vi "CreateSyslog.vi"(6 "timestamp":timestamp, 7 "type":T1, 8 "error in":errorcluster, 10 "executiontime":dbl, 11 "log":string) -> (0 "error out":errorcluster, 3 "syslog out":refnum<class "syslogs.lvclass">)   [LabVIEW 2020, in "ORM_Examples.lvlib" / "syslogs.lvclass"]
uses:
  syslogs.lvclass
  type.ctl
  syslogs.lvclass/syslogs.ctl
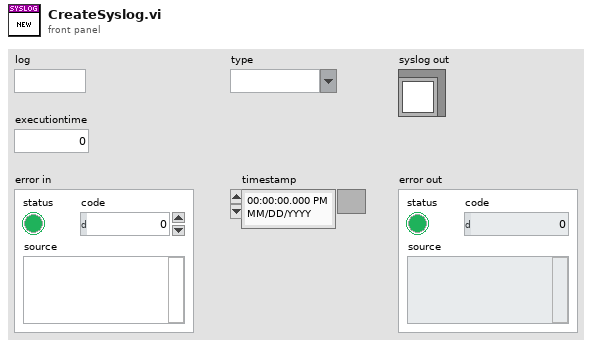
[diagram p1: front panel]
types:
  T1 = typedef "ORM_Examples.lvlib/syslogs.lvclass/type.ctl" = string
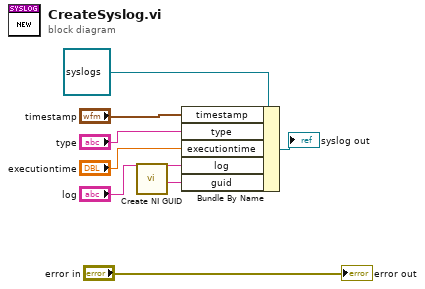
[diagram p0: block diagram]
diagram:
  n1 = call <vilib>:"Create NI GUID.vi"() -> ("NI GUID"=w1:string)
  n2 = Bundle By Name(cluster=refnum<class "syslogs.lvclass"> refnum ("ORM_Examples.lvlib:syslogs.lvclass"), "timestamp"="timestamp", "type"="type", "executiontime"="executiontime", "log"="log", "guid"=w1) -> (→"syslog out":refnum<class "syslogs.lvclass">)
  "error out" <- "error in"
